vi "Python Interoperation Example.vi"() -> ()   [LabVIEW 2020]
uses:
  LabVIEW/g_ar_toolkit.image/NewImageARGBArray.vi
  LabVIEW/g_ar_toolkit.image/DrawImageToPictureARGB.vi
  LabVIEW/g_ar_toolkit.image/DrawImageToPictureARGB.vi/8cd07b1b-062e-4fe4-9e87-2eb3dc89fe0e.vi
  LabVIEW/g_ar_toolkit.common/Module Path.vi
  <vilib>/Utility/error.llb/Error Cluster From Error Code.vi
  LabVIEW/g_ar_toolkit.image/g_ar_toolkit.image.lvlib
panel:
  out "error out":errorcluster
  out "Picture":picture
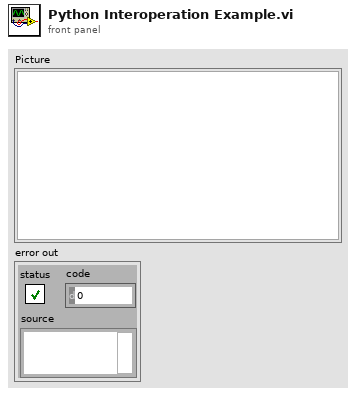
[diagram p1: front panel]
types:
  T1 = typedef "g_ar_toolkit.image.lvlib/ARGB Image.ctl" = refnum<data-value>
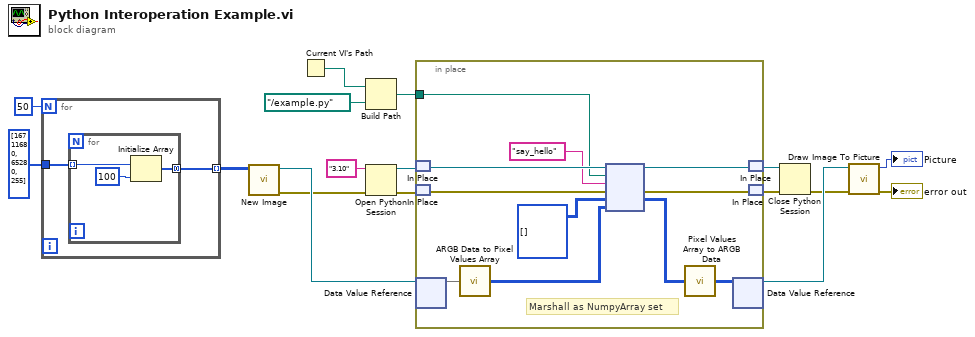
[diagram p0: block diagram]
diagram:
  n1 = for {
    N: 50 -> [_]
    tunnel: u32[] [16711680, 65280, 255] ("color(black)") -> [w19]
    tunnel: [w18] -> w5 mode=indexing
    n2 = for {
      tunnel: w19 -> [w22] mode=indexing
      tunnel: [w20] -> w18 mode=concatenating
      n3 = Initialize Array(w22, 100 ("dimension size")) -> (w20:u32[])
    }
  }
  n4 = call-poly "New Image.vi"("U32 ARBG Data  (Default: Empty)"=w5) -> ("error out"=w4:errorcluster, "New ARGB Image"=w12:T1)  [unwired: 9 in]
  n5 = Current VI's Path() -> (path=w6:path)
  n6 = Build Path(base path=w6, name or relative path=path "../example.py" ("module path")) -> (appended path=w8:path)
  n7 = Open Python Session(python version="3.10" ("Python version"), 3:w4) -> (session out=w2:refnum<k35>, error out=w3:errorcluster)  [unwired: 1 in]
  n8 = in-place {
    in-place-border: w8 -> [w25]
    # "Marshall as NumpyArray set"
    n9 = in-place-match #1(w2) -> (w33:refnum<k35>)
    n10 = in-place-match #2(w3) -> (w24:errorcluster)
    n11 = in-place-dvr #3(w12) -> (w30:u32[][])  [unwired: 1 out]
    n12 = call "ARGB Data to Pixel Values Array.vi"("ARGB Data"=w30) -> ("Pixel Values"=w29:u8[][][])
    n13 = node(w33, w25, "say_hello" ("function name"), w24, u8[][][] [] ("Pixel Values"), w29) -> (w32:refnum<k35>, w23:errorcluster, w26:u8[][][])  [unwired: 1 in, 2 out]
    n14 = call "Pixel Values Array to ARGB Data.vi"("Pixel Values"=w26) -> ("ARGB Data"=w28:u32[][])
    n15 = in-place-dvr #3(w28) -> (w14:T1)  [unwired: 1 out]
    n16 = in-place-match #1(w32) -> (w15:refnum<k35>)
    n17 = in-place-match #2(w23) -> (w7:errorcluster)
  }
  n18 = Close Python Session(session in=w15, error in=w7) -> (11:w11:errorcluster)
  n19 = call-poly "Draw Image To Picture.vi"("error in (no error)"=w11, "ARGB Image Source"=w14) -> ("error out"=→"error out":errorcluster, "Picture"=→"Picture":picture)  [unwired: 8 in]
